vi "Create Report (Template).vi"(8 "error in (no error)":errorcluster, 10 "Report Path":path, 11 "Test Report.Default in":refnum<class "Test Report.Template.lvclass">) -> (0 "error out":errorcluster, 3 "Test Report.Default out":refnum<class "Test Report.Template.lvclass">)   [LabVIEW 2013, in "Caraya.lvlib" / "Test Report.Template.lvclass"]
uses:
  Test Report.Template.lvclass
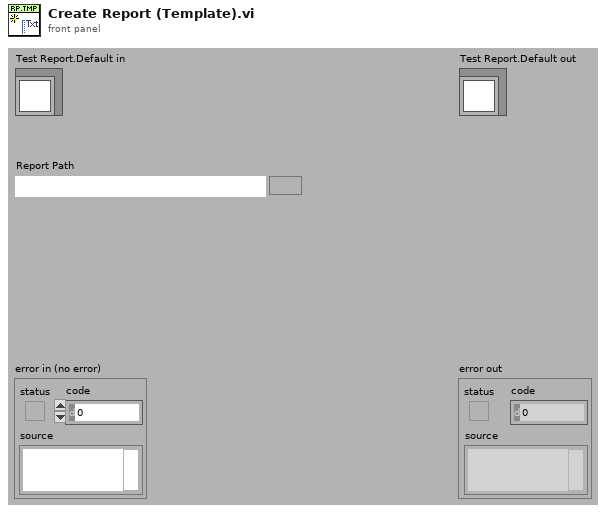
[diagram p1: front panel]
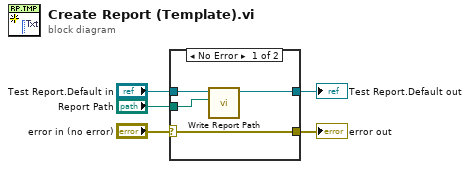
[diagram p0: block diagram]
diagram:
  n1 = case shown="No Error" "error in (no error)" {
    selector: "error in (no error)" -> [w6 w10]
    tunnel: "Test Report.Default in" -> [w9 w11]
    tunnel: [w8 w11] -> w4
    tunnel: "Report Path" -> [w7 _]
    tunnel: [w6 w10] -> w1
    frame No Error {
      n2 = call "Write Report Path.vi"("Report Path"=w7, "Test Report.Default in"=w9) -> ("Test Report.Default out"=w8:refnum<class "Test Report.Template.lvclass">)  [unwired: 9 in]
    }
    frame Error {
    }
  }
  "error out" <- w1
  "Test Report.Default out" <- w4
